vi "xiUtils - Elapsed Time - HighRes.vi"(8 "error in (no error)":errorcluster, 11 "Tick (ms) In":dbl) -> (0 "error out":errorcluster, 1 "Elapsed Time(ms)":dbl, 3 "Tick (ms) Out":dbl)   [LabVIEW 2018]
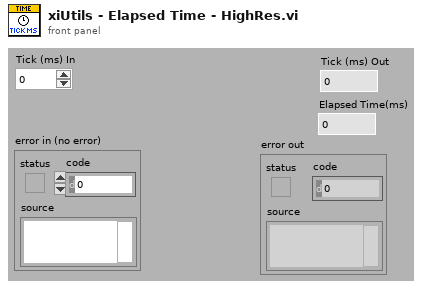
[diagram p1: front panel]
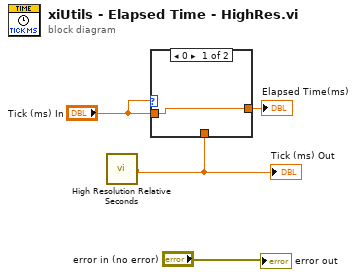
[diagram p0: block diagram]
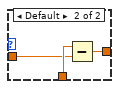
[diagram p2: hidden frame]
diagram:
  n1 = call <vilib>:"High Resolution Relative Seconds.vi"() -> ("relative seconds"=w2:dbl)
  "Tick (ms) Out" <- w2
  n2 = case shown="0" "Tick (ms) In" {
    tunnel: w2 -> [_ w8]
    tunnel: [w5 w7] -> w4
    tunnel: "Tick (ms) In" -> [w5 w6]
    frame 0 {
    }
    frame Default {
      n3 = Subtract(x=w8, y=w6) -> (x-y=w7:dbl)
    }
  }
  "Elapsed Time(ms)" <- w4
  "error out" <- "error in (no error)"
